vi "Read Instrument 3.lvclass.vi"(8 "error in (no error)":errorcluster, 11 "Measurement3D in":refnum<class "Measurement3D.lvclass">) -> (0 "error out":errorcluster, 2 "Instrument.lvclass":refnum<class "Instrument.lvclass">, 3 "Measurement3D out":refnum<class "Measurement3D.lvclass">)   [LabVIEW 2014, in "Measurement3D.lvclass"]
uses:
  Measurement3D.lvclass
  Instrument/Instrument/Instrument.lvclass
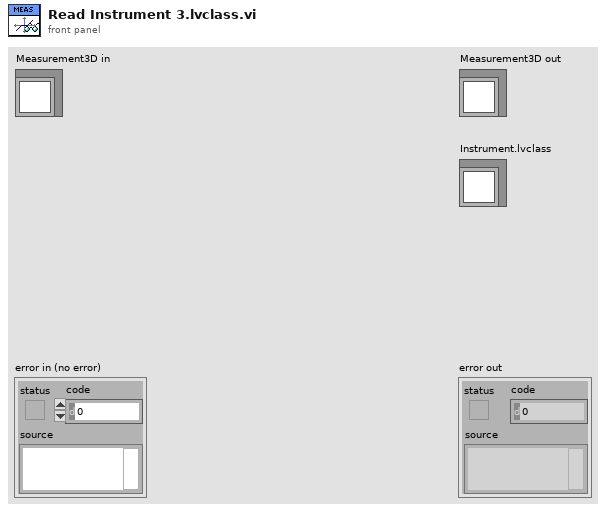
[diagram p1: front panel]
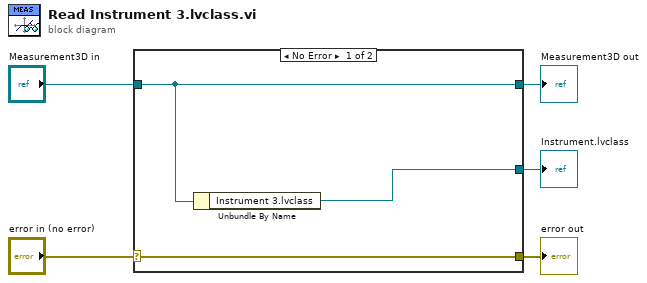
[diagram p0: block diagram]
diagram:
  n1 = case shown="No Error" "error in (no error)" {
    selector: "error in (no error)" -> [w8 w9]
    tunnel: [w8 w9] -> w4
    tunnel: [w7 w10] -> w2
    tunnel: "Measurement3D in" -> [w7 w10]
    tunnel: [w6 _] -> w1
    frame No Error {
      n2 = Unbundle By Name(w7) -> ("Instrument 3.lvclass"=w6:refnum<class "Instrument.lvclass">)
    }
    frame Error {
    }
  }
  "error out" <- w4
  "Measurement3D out" <- w2
  "Instrument.lvclass" <- w1
